vi "4461 - Create Reference Waveforms.vi"(6 "time delay":dbl, 8 "error in (no error)":errorcluster, 9 "sampling info":cluster{"Fs":dbl, "#s":dbl}={"Fs"=1000.0, "#s"=1000.0} {"Fs" format="%.2p"}, 10 "reset signal":bool, 11 "Lockin":T1={"REF f (Hz)"=[13.0, 13.0, 13.0, 13.0, 13.0, 13.0, 13.0, 13.0], "REF phi (deg)"=[0.0, 0.0, 0.0, 0.0, 0.0, 0.0, 0.0, 0.0]} {"REF phi (deg)" format="%#_3g"}) -> (0 "error out":errorcluster, 1 "phase out":dbl[](array[numeric]), 2 "AO Array":waveform(dbl)[](array[waveform]), 3 "Lockin 2":T1={"REF f (Hz)"=[13.0, 13.0, 13.0, 13.0, 13.0, 13.0, 13.0, 13.0], "REF phi (deg)"=[0.0, 0.0, 0.0, 0.0, 0.0, 0.0, 0.0, 0.0]} {"REF phi (deg)" format="%#_3g"})   [LabVIEW 2016]
uses:
  <vilib>/Analysis/2dsp.llb/Decimate (single shot).vi
  <vilib>/Analysis/2dsp.llb/Decimate (single shot, DBL).vi
  <vilib>/Utility/error.llb/Error Cluster From Error Code.vi
  <vilib>/measure/NI_MABase.lvlib
panel:
  out "Waveform Graph 2":waveform(dbl)[](graph)
  out "Numeric":i32
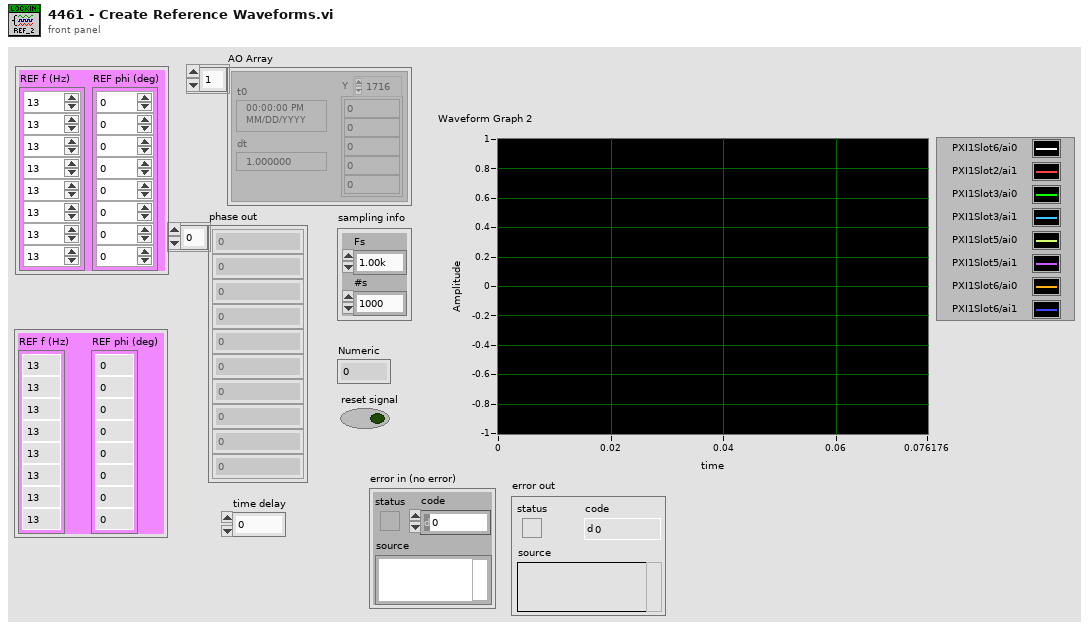
[diagram p1: front panel]
types:
  T1 = cluster{"REF f (Hz)":dbl[], "REF phi (deg)":dbl[]}
  T2 = enum16{"Sine Wave", "Triangle Wave", "Square Wave", "Sawtooth Wave"}
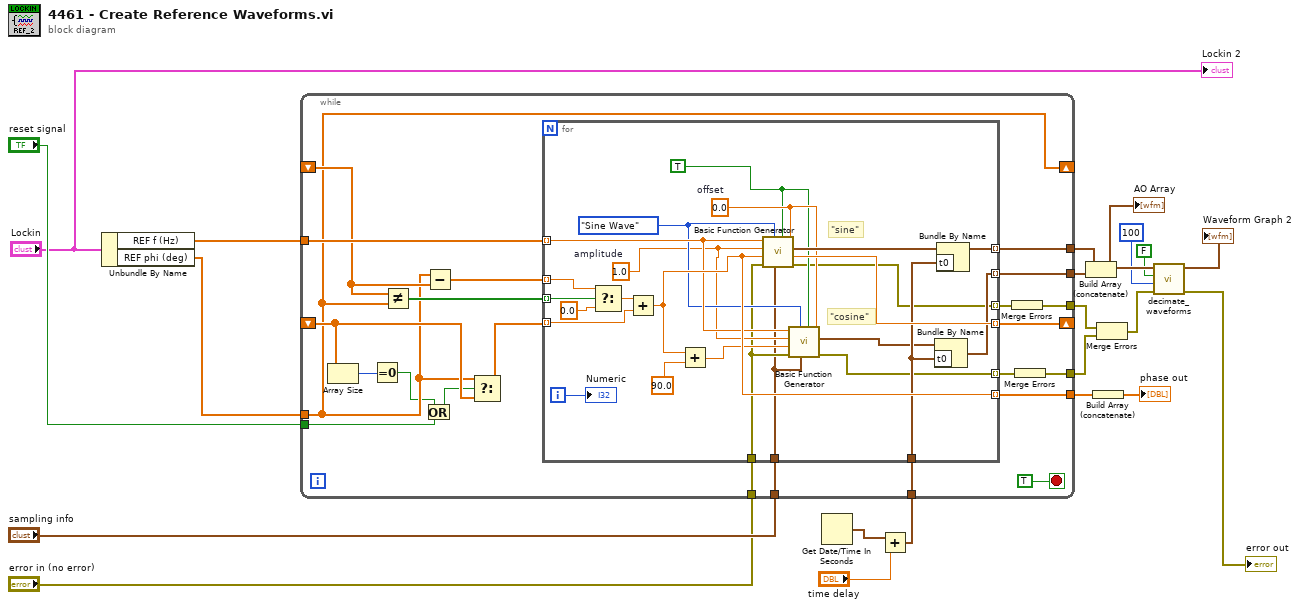
[diagram p0: block diagram]
diagram:
  n1 = Unbundle By Name("Lockin") -> ("REF f (Hz)"=w14:dbl[], "REF phi (deg)"=w3:dbl[])
  n2 = Get Date/Time In Seconds() -> (seconds since 1Jan1904=w20:timestamp)
  n3 = Add(x=w20, y="time delay") -> (x+y=w5:timestamp)
  n4 = while {
    tunnel: "sampling info" -> [w44]
    tunnel: [w43] -> w15
    tunnel: w3 -> [w32]
    tunnel: w14 -> [w42]
    shift-right: [w32] -> _
    shift-left: _ -> [w39]
    shift-right: [w37] -> _
    shift-left: _ -> [w34]
    tunnel: w5 -> [w35]
    tunnel: "reset signal" -> [w29]
    tunnel: [w28] -> w18
    tunnel: [w27] -> w16
    tunnel: "error in (no error)" -> [w26]
    tunnel: [w24] -> w8
    tunnel: [w22] -> w9
    stop <- TRUE stop-if-true
    n5 = Array Size(array=w34) -> (size(s)=w33:i32)
    n6 = Equal To 0?(x=w33) -> (x = 0?=w30:bool)
    n7 = Not Equal?(x=w39, y=w32) -> (x != y?=w40:bool[])
    n8 = Or(x=w30, y=w29) -> (x .or. y?=w31:bool)
    n9 = Subtract(x=w32, y=w39) -> (x-y=w38:dbl[])
    n10 = Select(t=w32, s=w31, f=w34) -> (s? t:f=w36:dbl[])
    n11 = for {
      tunnel: w42 -> [w56] mode=indexing
      tunnel: [w67] -> w43 mode=indexing
      tunnel: w44 -> [w47]
      tunnel: w40 -> [w61] mode=indexing
      tunnel: w38 -> [w63] mode=indexing
      tunnel: [w59] -> w37 mode=indexing
      tunnel: w36 -> [w64] mode=indexing
      tunnel: w35 -> [w55]
      tunnel: [w58] -> w28 mode=indexing
      tunnel: [w53] -> w27 mode=indexing
      tunnel: w26 -> [w48]
      tunnel: [w46] -> w25 mode=indexing
      tunnel: [w45] -> w23 mode=indexing
      i -> [w60]
      w49 = TRUE ("reset signal")
      w51 = 0.0  # offset
      w52 = T2."Sine Wave" ("signal type")
      w50 = 1.0  # amplitude
      # "\"cosine\""
      # "\"sine\""
      n12 = Select(t=w63, s=w61, f=0.0) -> (s? t:f=w65:dbl)
      n13 = Add(x=w65, y=w64) -> (x+y=w58:dbl)
      n14 = Add(x=w58, y=90.0) -> (x+y=w57:dbl)
      n15 = call <vilib>:"Basic Function Generator.vi"("offset"=w51, "reset signal"=w49, "sampling info"=w47, "signal type"=w52, "error in (no error)"=w48, "phase"=w58, "amplitude"=w50, "frequency"=w56) -> ("error out"=w46:errorcluster, "phase out"=w59:dbl, "signal out"=w68:waveform(dbl))  [unwired: 1 in]
      n16 = call <vilib>:"Basic Function Generator.vi"("offset"=w51, "reset signal"=w49, "sampling info"=w47, "signal type"=w52, "error in (no error)"=w48, "phase"=w57, "amplitude"=w50, "frequency"=w56) -> ("error out"=w45:errorcluster, "signal out"=w54:waveform(dbl))  [unwired: 1 in, 1 out]
      n17 = Bundle By Name(cluster=w54, "t0"=w55) -> (w53:waveform(dbl))
      n18 = Bundle By Name(cluster=w68, "t0"=w55) -> (w67:waveform(dbl))
      "Numeric" <- w60
    }
    n19 = Merge Errors(w25) -> (w24:errorcluster)
    n20 = Merge Errors(w23) -> (w22:errorcluster)
  }
  n21 = Build Array (concatenate)(w15, w16) -> (w11:waveform(dbl)[])
  "AO Array" <- w11
  n22 = Build Array (concatenate)(w18) -> (→"phase out":dbl[])
  n23 = Merge Errors(w8, w9) -> (w7:errorcluster)
  n24 = call "decimate_waveforms.vi"("Input Signal"=w11, "averaging"=FALSE, "decimating factor"=100, "error in (no error)"=w7) -> ("Decimated Waveforms"=→"Waveform Graph 2":waveform(dbl)[], "error out"=→"error out":errorcluster)  [unwired: 5 in]
  "Lockin 2" <- "Lockin"
